vi "tank.vi"() -> ()   [LabVIEW 2020]
panel:
  in  "stop":bool
  out "Tank":dbl(slide) scale=0.0..100.0
  in  "Level":dbl(slide) scale=0.0..100.0
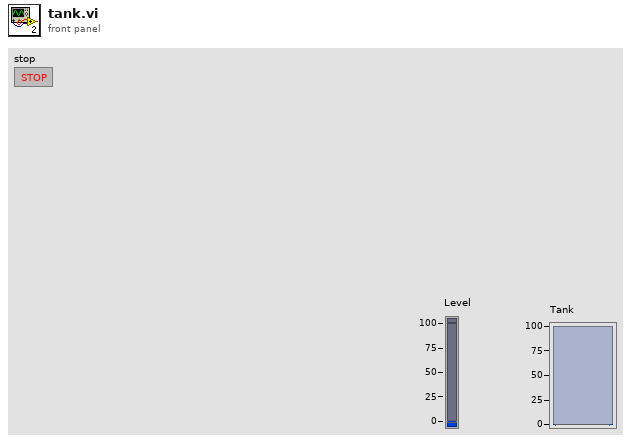
[diagram p1: front panel]
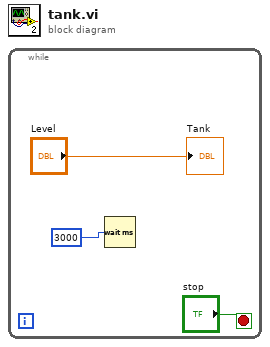
[diagram p0: block diagram]
diagram:
  n1 = while {
    stop <- "stop" stop-if-true
    n2 = Wait (ms)(milliseconds to wait=u32 3000 ("millisecond timer value")) -> ()  [unwired: 1 out]
    "Tank" <- "Level"
  }
